vi "工位1运行.vi"(11 "簇":T2={"工位1"=refnum, "1-3参数设置"=refnum, "总时间"=0, "NG？"=FALSE, "循环次数"=0, "步骤次数"=0, "单个时间"=0, "完成?"=FALSE, "路径"=path "e:/LDM数据/工位一", "1"=19, "2"=19, "3"=19, "4"=19, "AI"=24, "范围"=24, "保存间隔时间"=1} {"保存间隔时间" min=1 step=1}) -> (3 "簇 2":T2={"工位1"=refnum, "1-3参数设置"=refnum, "总时间"=0, "NG？"=FALSE, "循环次数"=0, "步骤次数"=0, "单个时间"=0, "完成?"=FALSE, "路径"=path "e:/LDM数据/工位一", "1"=19, "2"=19, "3"=19, "4"=19, "AI"=24, "范围"=24, "保存间隔时间"=1} {"保存间隔时间" min=1 step=1})   [LabVIEW 2012]
uses:
  <vilib>/ptbypt/NI_PtbyPt.lvlib
panel:
  in  "1":T1 {"设定循环次数  5" min=0.0 format="%#.2f"; "已用时间  9" min=0.0 format="%#.2f"; "运行总时间  8" min=0.0 format="%#.2f"; "当前步骤运行时间 7" min=0.0 format="%#.2f"; "当前次数 6" min=0.0 format="%#.2f"; "1-1 5"."运行时间" min=0.0 format="%#.2f"; "1-1 4"."运行时间" min=0.0 format="%#.2f"; "1-1 3"."运行时间" min=0.0 format="%#.2f"; "1-1 2"."运行时间" min=0.0 format="%#.2f"; "1-1"."运行时间" min=0.0 format="%#.2f"}
  # "启用"
  # "min"
  # "启用"
  # "min"
  # "启用"
  # "min"
  # "启用"
  # "min"
  # "启用"
  # "min"
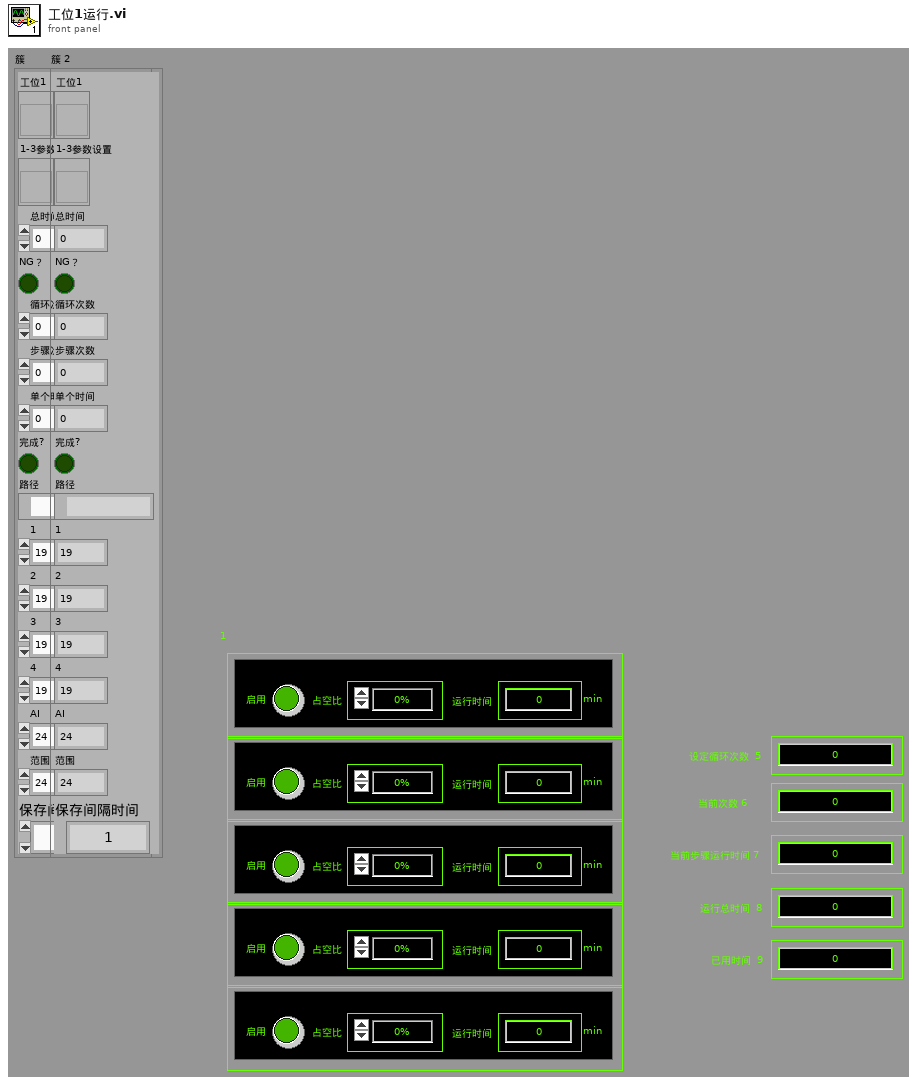
[diagram p1: front panel]
types:
  T1 = cluster{"1-1":cluster{bool, "占空比":enum16{"0%", "28%", "100%"}, "运行时间":dbl}, "1-1 2":cluster{bool, "占空比":enum16{"0%", "28%", "100%"}, "运行时间":dbl}, "1-1 3":cluster{bool, "占空比":enum16{"0%", "28%", "100%"}, "运行时间":dbl}, "1-1 4":cluster{bool, "占空比":enum16{"0%", "28%", "100%"}, "运行时间":dbl}, "1-1 5":cluster{bool, "占空比":enum16{"0%", "28%", "100%"}, "运行时间":dbl}, "设定循环次数  5":dbl, "当前次数 6    ":dbl, "当前步骤运行时间 7":dbl, "运行总时间  8":dbl, "已用时间  9":dbl}
  T2 = typedef "控件 4.ctl" = cluster{"工位1":refnum<vi>, "1-3参数设置":refnum<vi>, "总时间":u32, "NG？":bool, "循环次数":i32, "步骤次数":i32, "单个时间":u32, "完成?":bool, "路径":path, "1":i32, "2":i32, "3":i32, "4":i32, "AI":i32, "范围":i32, "保存间隔时间":u64}
  T3 = typedef "控件 3.ctl" = enum16{"初始化", "读取", "写入", "退出"}
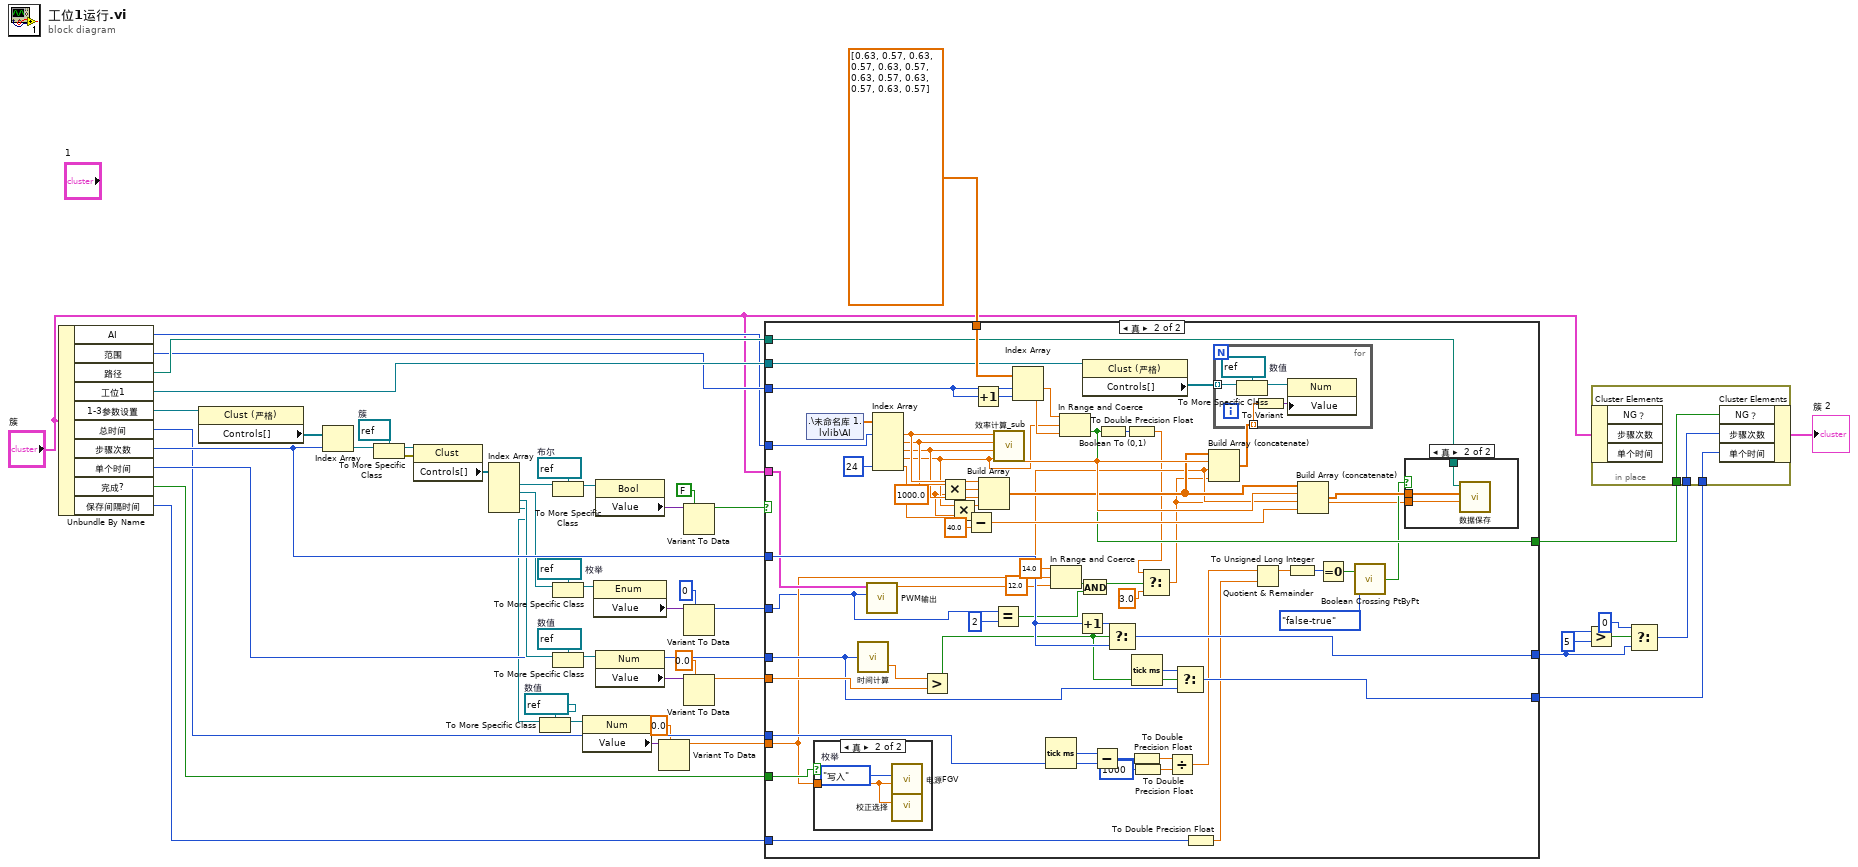
[diagram p0: block diagram]
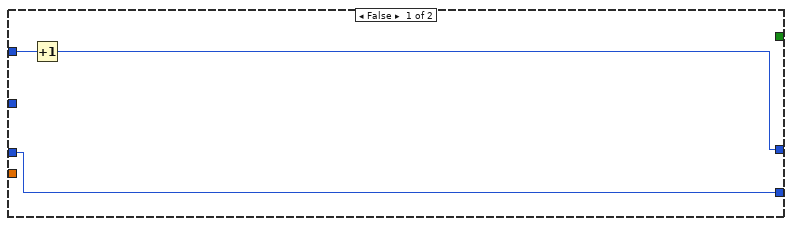
[diagram p2: hidden frame]
diagram:
  w20 = refnum<vi> refnum  # 数值
  w28 = refnum<vi> refnum  # 数值
  w35 = refnum<vi> refnum  # 枚举
  w41 = refnum<vi> refnum  # 布尔
  w47 = refnum<vi> refnum  # 簇
  n1 = Unbundle By Name("簇") -> ("AI"=w4:i32, "范围"=w5:i32, "路径"=w6:path, "工位1"=w49:refnum<vi>, "1-3参数设置"=w48:refnum<vi>, "总时间"=w23:u32, "步骤次数"=w37:i32, "单个时间"=w24:u32, "完成?"=w2:bool, "保存间隔时间"=w1:u64)
  n2 = property class="Clust (严格)"(reference=w48) -> ("Controls[]"=w14:refnum<vi>[])  [unwired: 1 in, 2 out]
  n3 = Index Array(array=w14, index=w37) -> (element=w46:refnum<vi>)
  n4 = To More Specific Class(target class=w47, reference=w46) -> (specific class reference=w45:refnum<vi>, error out=w44:errorcluster)  [unwired: 1 in]
  n5 = property class="Clust"(reference=w45, error in=w44) -> ("Controls[]"=w43:refnum<vi>[])  [unwired: 2 out]
  n6 = Index Array(array=w43) -> (element #1=w38:refnum<vi>, element #2=w33:refnum<vi>, element #3=w26:refnum<vi>, element #4=w16:refnum<vi>)  [unwired: 4 in]
  n7 = To More Specific Class(target class=w20, reference=w16) -> (specific class reference=w18:refnum<vi>)  [unwired: 1 in, 1 out]
  n8 = To More Specific Class(target class=w41, reference=w38) -> (specific class reference=w42:refnum<vi>)  [unwired: 1 in, 1 out]
  n9 = To More Specific Class(target class=w35, reference=w33) -> (specific class reference=w34:refnum<vi>)  [unwired: 1 in, 1 out]
  n10 = To More Specific Class(target class=w28, reference=w26) -> (specific class reference=w29:refnum<vi>)  [unwired: 1 in, 1 out]
  n11 = property class="Num"(reference=w18) -> ("Value"=w17:variant)  [unwired: 1 in, 2 out]
  n12 = property class="Enum"(reference=w34) -> ("Value"=w36:variant)  [unwired: 1 in, 2 out]
  n13 = property class="Bool"(reference=w42) -> ("Value"=w40:variant)  [unwired: 1 in, 2 out]
  n14 = property class="Num"(reference=w29) -> ("Value"=w27:variant)  [unwired: 1 in, 2 out]
  n15 = Variant To Data(type=0.0 ("步骤次数"), Variant=w17) -> (data=w7:dbl)  [unwired: 1 in, 1 out]
  n16 = Variant To Data(type=FALSE, Variant=w40) -> (data=w15:bool)  [unwired: 1 in, 1 out]
  n17 = Variant To Data(type=u16 0 ("步骤次数"), Variant=w36) -> (data=w31:u16)  [unwired: 1 in, 1 out]
  n18 = Variant To Data(type=0.0 ("步骤次数"), Variant=w27) -> (data=w25:dbl)  [unwired: 1 in, 1 out]
  n19 = case shown="真" w15 {
    tunnel: dbl[] [0.63, 0.57, 0.63, 0.57, 0.63, 0.57, 0.63, 0.57, 0.63, 0.57, 0.63, 0.57] -> [_ w117]
    tunnel: w49 -> [_ w116]
    tunnel: w37 -> [w53 w96]
    tunnel: w31 -> [_ w57]
    tunnel: w25 -> [_ w89]
    tunnel: w24 -> [w51 w87]
    tunnel: w23 -> [_ w72]
    tunnel: [_ w95] -> w22
    tunnel: [w52 w85] -> w9
    tunnel: [w51 w84] -> w13
    tunnel: w7 -> [_ w62]
    tunnel: w6 -> [_ w83]
    tunnel: w5 -> [_ w82]
    tunnel: w4 -> [_ w80]
    tunnel: "簇" -> [_ w79]
    tunnel: w2 -> [_ w78]
    tunnel: w1 -> [_ w66]
    frame False {
      n20 = Increment(x=w53) -> (x+1=w52:i32)
    }
    frame True {
      w67 = 1000.0 ("y")
      n21 = shared-variable ".\\未命名库 1.lvlib\\AI"() -> (w115:dbl[])  [unwired: 1 in, 1 out]
      n22 = case shown="真" w78 {
        tunnel: w62 -> [_ w118]
        frame False {
        }
        frame True {
          w119 = 控件_3."写入"  # 枚举
          n23 = call "电源FGV.vi"("Voltage"=w118, "枚举"=w119) -> ()  [unwired: 8 in, 2 out]
          n24 = call "校正选择.vi"("数值"=w118) -> ()  [unwired: 11 in]
        }
      }
      n25 = call "时间计算.vi"("跳变时间"=w87) -> ("数值"=w98:dbl)  [unwired: 1 out]
      n26 = call "PWM输出.vi"("步骤次数输入"=w57, "簇"=w79) -> ("步骤次数输出"=w90:dbl)  [unwired: 9 in]
      n27 = Index Array(array=w115, index #1=w80, index #5=24 ("索引")) -> (element #1=w107:dbl, element #2=w106:dbl, element #3=w105:dbl, element #4=w104:dbl, element #5=w100:dbl)  [unwired: 3 in]
      n28 = Greater?(x=w98, y=w89) -> (0:w88:bool)
      n29 = Multiply(x=w106, y=w67) -> (x*y=w69:dbl)
      n30 = Multiply(x=w104, y=w67) -> (x*y=w68:dbl)
      n31 = Subtract(x=w100, y=40.0) -> (x-y=w99:dbl)
      n32 = Increment(x=w82) -> (x+1=w81:i32)
      n33 = Build Array(w107, w69, w105, w68) -> (w103:dbl[])
      n34 = Equal?(x=w57, y=u16 2) -> (x = y?=w54:bool)
      n35 = call "效率计算_sub.vi"("输出电流"=w104, "输出电压"=w105, "输入电流"=w106, "输入电压"=w107) -> ("效率"=w109:dbl)  [unwired: 7 in]
      n36 = Index Array(array=w117, index #1=w82, index #2=w81) -> (element #1=w114:dbl, element #2=w113:dbl)
      n37 = Tick Count (ms)() -> (millisecond timer value=w77:u32)
      n38 = In Range and Coerce(upper limit=14.0 ("上限"), x=w62, lower limit=12.0 ("下限")) -> (In Range?=w61:bool)  [unwired: 1 out]
      n39 = In Range and Coerce(upper limit=w114, x=w104, lower limit=w113) -> (In Range?=w95:bool)  [unwired: 1 out]
      n40 = Increment(x=w96) -> (x+1=w97:i32)
      n41 = And(x=w61, y=w54) -> (x .and. y?=w55:bool)
      n42 = property class="Clust (严格)"(reference=w116) -> ("Controls[]"=w111:refnum<vi>[])  [unwired: 1 in, 2 out]
      n43 = Subtract(x=w77, y=w72) -> (x-y=w76:u32)
      n44 = Boolean To (0,1)(Boolean=w95) -> (0, 1=w112:i16)
      n45 = Select(t=w97, s=w88, f=w96) -> (s? t:f=w85:i32)
      n46 = To Double Precision Float(number=w112) -> (double precision float=w59:dbl)
      n47 = Tick Count (ms)() -> (millisecond timer value=w86:u32)
      n48 = To Double Precision Float(number=w76) -> (double precision float=w74:dbl)
      n49 = To Double Precision Float(number=u32 1000 ("y")) -> (double precision float=w73:dbl)
      n50 = Select(t=w59, s=w55, f=3.0 ("t")) -> (s? t:f=w60:dbl)
      n51 = Divide(x=w74, y=w73) -> (x/y=w71:dbl)
      n52 = Select(t=w86, s=w88, f=w87) -> (s? t:f=w84:u32)
      n53 = To Double Precision Float(number=w66) -> (double precision float=w65:dbl)
      n54 = Build Array (concatenate)(w103, w109, w90, w60) -> (w110:dbl[])
      n55 = for {
        tunnel: w111 -> [w127] mode=indexing
        tunnel: w110 -> [w124] mode=indexing
        w125 = refnum<vi> refnum  # 数值
        n56 = To More Specific Class(target class=w125, reference=w127) -> (specific class reference=w126:refnum<vi>)  [unwired: 1 in, 1 out]
        n57 = To Variant(anything=w124) -> (Variant=w123:variant)
        n58 = property class="Num"(reference=w126, "Value"=w123) -> ()  [unwired: 1 in, 2 out]
      }
      n59 = Quotient & Remainder(x=w71, y=w65) -> (x-y*floor(x/y)=w94:dbl)  [unwired: 1 out]
      n60 = To Unsigned Long Integer(number=w94) -> (unsigned 32bit integer=w70:u32)
      n61 = Build Array (concatenate)(w103, w109, w90, w99) -> (w108:dbl[])
      n62 = Equal To 0?(x=w70) -> (x = 0?=w93:bool)
      n63 = call <vilib>:"Boolean Crossing PtByPt.vi"("direction"=enum16{"either", "false-true", "true-false"}."false-true", "input"=w93) -> ("crossing"=w91:bool)  [unwired: 1 in]
      n64 = case shown="真" w91 {
        tunnel: w60 -> [_ w122]
        tunnel: w108 -> [_ w121]
        tunnel: w83 -> [_ w120]
        frame False {
        }
        frame True {
          n65 = call "数据保存.vi"("数值"=w122, "数组"=w121, "appended path"=w120) -> ()  [unwired: 9 in]
        }
      }
    }
  }
  n66 = Greater?(x=w9, y=5) -> (0:w11:bool)
  n67 = Select(t=0 ("y"), s=w11, f=w9) -> (s? t:f=w8:i32)
  n68 = in-place {
    in-place-border: w22 -> [w130]
    in-place-border: w8 -> [w129]
    in-place-border: w13 -> [w128]
    n69 = in-place-cluster #1("簇") -> ()  [unwired: 3 out]
    n70 = in-place-cluster #1("NG？"=w130, "步骤次数"=w129, "单个时间"=w128) -> (→"簇 2":T2)
  }
